vi "Construct Shutdown Sink.vi"(11 "Stop Queue":refnum<queue>) -> (3 "Shutdown Sink out":refnum<class "Shutdown Sink.lvclass">)   [LabVIEW 2017, in "Network Sink.lvlib" / "Shutdown Sink.lvclass"]
uses:
  <vilib>/gpm_packages/@cs/event-logger/Source/Network Sink/Shutdown Sink/Shutdown Sink.lvclass
  <vilib>/gpm_packages/@cs/event-logger/Source/Network Sink/Shutdown Sink/Shutdown Sink.lvclass/Shutdown Sink.ctl
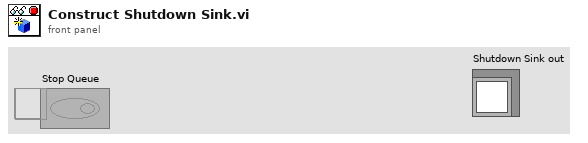
[diagram p1: front panel]
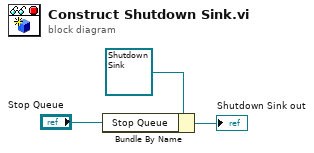
[diagram p0: block diagram]
diagram:
  n1 = Bundle By Name(cluster=refnum<class "Shutdown Sink.lvclass"> refnum ("Shutdown Sink in"), "Stop Queue"="Stop Queue") -> (→"Shutdown Sink out":refnum<class "Shutdown Sink.lvclass">)
